vi "ConvDecode.vi"(8 "error in (no error)":errorcluster, 10 "Encode Parameter":T1={"constraint length (K)"=3, "initial state"=0, "Encode factor"=0} {"initial state" format="%.0x"}, 11 "Input Bits":i8[](array[numeric])) -> (0 "error out":errorcluster, 3 "output bit stream":i8[](array[numeric]))   [LabVIEW 2014]
uses:
  <vilib>/addons/Modulation/Digital/Channel Coding/MT Convolutional Decoder (Viterbi Hard Decision, Rate).vi
  <vilib>/addons/Modulation/niDMT.lvlib
panel:
  out "size(s)":i32
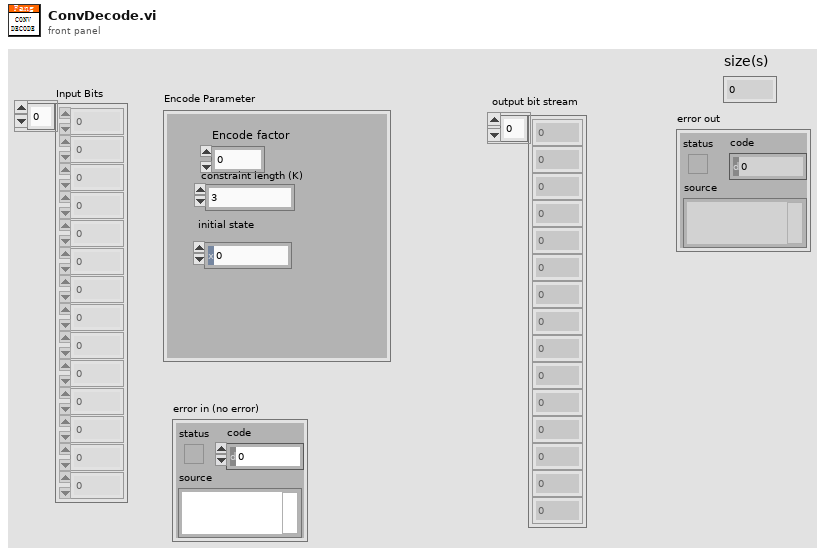
[diagram p1: front panel]
types:
  T1 = cluster{"constraint length (K)":i32, "initial state":u32, "Encode factor":i32}
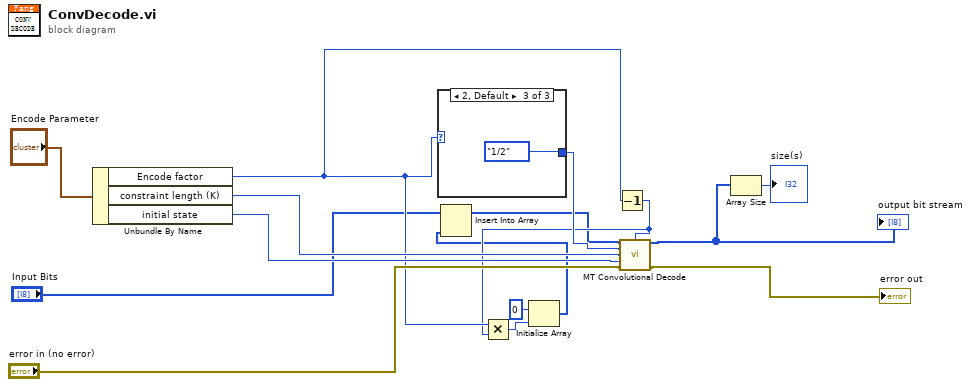
[diagram p0: block diagram]
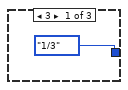
[diagram p2: hidden frame]
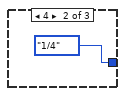
[diagram p3: hidden frame]
diagram:
  n1 = Unbundle By Name("Encode Parameter") -> ("Encode factor"=w6:i32, "constraint length (K)"=w11:i32, "initial state"=w12:u32)
  n2 = case shown="2, Default" w6 {
    tunnel: [enum16{"1/2", "1/3", "1/4", "2/3", "3/4"}."1/3" ("rate (k/n)") enum16{"1/2", "1/3", "1/4", "2/3", "3/4"}."1/4" ("rate (k/n)") enum16{"1/2", "1/3", "1/4", "2/3", "3/4"}."1/2" ("rate (k/n)")] -> w14
    frame 3 {
    }
    frame 4 {
    }
    frame 2, Default {
    }
  }
  n3 = Decrement(x=w6) -> (x-1=w5:i32)
  n4 = Multiply(x=w6, y=w5) -> (x*y=w7:i32)
  n5 = Initialize Array(i8 0 ("element"), w7) -> (w2:i8[])
  n6 = Insert Into Array(array="Input Bits", new element=w2) -> (w1:i8[])  [unwired: 1 in]
  n7 = call-poly <vilib>:"MT Convolutional Decode.vi"("input bit stream"=w1, "traceback depth (D)"=w5, "rate (k/n)"=w14, "constraint length (K)"=w11, "initial state"=w12, "error in (no error)"="error in (no error)") -> ("output bit stream"=w9:i8[], "error out"=→"error out":errorcluster)  [unwired: 7 in, 1 out]
  "output bit stream" <- w9
  n8 = Array Size(array=w9) -> (size(s)=→"size(s)":i32)
